vi "ql2_term_to_id.vi"(11 "term_type":T1) -> (2 "term_type_ids":u32[](array[numeric]), 3 "id":u32)   [LabVIEW 2017, in "rethinkdb.lvlib"]
uses:
  rethinkdb.lvlib
  ql2_term.ctl
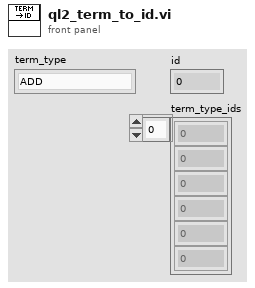
[diagram p1: front panel]
types:
  T1 = typedef "rethinkdb.lvlib/ql2_term.ctl" = enum8{"ADD", "AND", "APPEND", "APRIL", "ARGS", "ASC", "AUGUST", "AVG", "BETWEEN", "BETWEEN_DEPRECATED", "BINARY", "BIT_AND", "BIT_NOT", "BIT_OR", "BIT_SAL", "BIT_SAR", "BIT_XOR", "BRACKET", "BRANCH", "CEIL", "CHANGES", "CHANGE_AT", "CIRCLE", "COERCE_TO", "CONCAT_MAP", "CONFIG", "CONTAINS", "COUNT", "DATE", "DATUM", "DAY", "DAY_OF_WEEK", "DAY_OF_YEAR", "DB", "DB_CREATE", "DB_DROP", "DB_LIST", "DECEMBER", "DEFAULT", "DELETE", "DELETE_AT", "DESC", "DIFFERENCE", "DISTANCE", "DISTINCT", "DIV", "DOWNCASE", "DURING", "EPOCH_TIME", "EQ", "EQ_JOIN", "ERROR", "FEBRUARY", "FILL", "FILTER", "FLOOR", "FOLD", "FOR_EACH", "FRIDAY", "FUNC", "FUNCALL", "GE", "GEOJSON", "GET", "GET_ALL", "GET_FIELD", "GET_INTERSECTING", "GET_NEAREST", "GET_WRITE_HOOK", "GRANT", "GROUP", "GT", "HAS_FIELDS", "HOURS", "HTTP", "IMPLICIT_VAR", "INCLUDES", "INDEX_CREATE", "INDEX_DROP", "INDEX_LIST", "INDEX_RENAME", "INDEX_STATUS", "INDEX_WAIT", "INFO", "INNER_JOIN", "INSERT", "INSERT_AT", "INTERSECTS", "IN_TIMEZONE", "ISO8601", "IS_EMPTY", "JANUARY", "JAVASCRIPT", "JSON", "JULY", "JUNE", "KEYS", "LE", "LIMIT", "LINE", "LITERAL", "LT", "MAKE_ARRAY", "MAKE_OBJ", "MAP", "MARCH", "MATCH", "MAX", "MAXVAL", "MAY", "MERGE", "MIN", "MINUTES", "MINVAL", "MOD", "MONDAY", "MONTH", "MUL", "NE", "NOT", "NOVEMBER", "NOW", "NTH", "OBJECT", "OCTOBER", "OFFSETS_OF", "OR", "ORDER_BY", "OUTER_JOIN", "PLUCK", "POINT", "POLYGON", "POLYGON_SUB", "PREPEND", "RANDOM", "RANGE", "REBALANCE", "RECONFIGURE", "REDUCE", "REPLACE", "ROUND", "SAMPLE", "SATURDAY", "SECONDS", "SEPTEMBER", "SET_DIFFERENCE", "SET_INSERT", "SET_INTERSECTION", "SET_UNION", "SET_WRITE_HOOK", "SKIP", "SLICE", "SPLICE_AT", "SPLIT", "STATUS", "SUB", "SUM", "SUNDAY", "SYNC", "TABLE", "TABLE_CREATE", "TABLE_DROP", "TABLE_LIST", "THURSDAY", "TIME", "TIMEZONE", "TIME_OF_DAY", "TO_EPOCH_TIME", "TO_GEOJSON", "TO_ISO8601", "TO_JSON_STRING", "TUESDAY", "TYPE_OF", "UNGROUP", "UNION", "UPCASE", "UPDATE", "UUID", "VALUES", "VAR", "WAIT", "WEDNESDAY", "WITHOUT", "WITH_FIELDS", "YEAR", "ZIP", "invalid"}
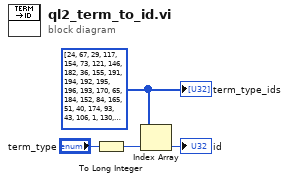
[diagram p0: block diagram]
diagram:
  w1 = u32[] [24, 67, 29, 117, 154, 73, 121, 146, 182, 36, 155, 191, 194, 192, 195, 196, 193, 170, 65, 184, 152, 84, 165, 51, 40, 174, 93, 43, 106, 1, 130, 131, 132, 14, 57, 58, 59, 125, 92, 54, 83, 74, 95, 162, 42, 27, 142, 105, 101, 17, 50, 12, 115, 167, 39, 183, 187, 68, 111, 69, 64, 22, 157, 16, 78, 31, 166, 168, 190, 188, 144, 21, 32, 133, 153, 13, 164, 75, 76, 77, 156, 139, 140, 79, 48, 56, 82, 163, 104, 99, 86, 114, 11, 98, 120, 119, 94, 20, 71, 160, 137, 19, 2, 3, 38, 116, 97, 148, 181, 118, 35, 147, 134, 180, 28, 107, 129, 26, 18, 23, 124, 103, 45, 143, 123, 87, 66, 41, 49, 33, 159, 161, 171, 80, 151, 173, 179, 176, 37, 55, 185, 81, 112, 135, 122, 91, 88, 89, 90, 189, 70, 30, 85, 149, 175, 25, 145, 113, 138, 15, 60, 61, 62, 110, 136, 127, 126, 102, 158, 100, 172, 108, 52, 150, 44, 141, 53, 169, 186, 10, 177, 109, 34, 96, 128, 72] ("ids")
  n1 = To Long Integer(number="term_type") -> (32bit integer=w3:i32)
  n2 = Index Array(array=w1, index=w3) -> (element=→"id":u32)
  "term_type_ids" <- w1
